vi "niRFUtil MASMT Util Constrained Linear Fit (SGL).vi"(0 "Y":sgl[](array[numeric]), 1 "method":i32(ring) items=["Least Square", "Least Absolute Residual", "Bisquare"], 5 "X":sgl[](array[numeric]), 7 "Weight":sgl[](array[numeric]), 9 "tolerance":sgl=0.0001, 11 "error in (no error)":errorcluster, 12 "parameter bounds":T1={"slope min"=-inf, "slope max"=inf, "intercept min"=-inf, "intercept max"=inf}) -> (4 "Best Linear Fit":sgl[](array[numeric]), 6 "slope":sgl, 8 "intercept":sgl, 10 "residue":sgl, 15 "error out":errorcluster)   [LabVIEW 2015, in "niRFUtil.lvlib"]
uses:
  niRFUtil.lvlib
  <vilib>/Analysis/NI_AALPro.lvlib
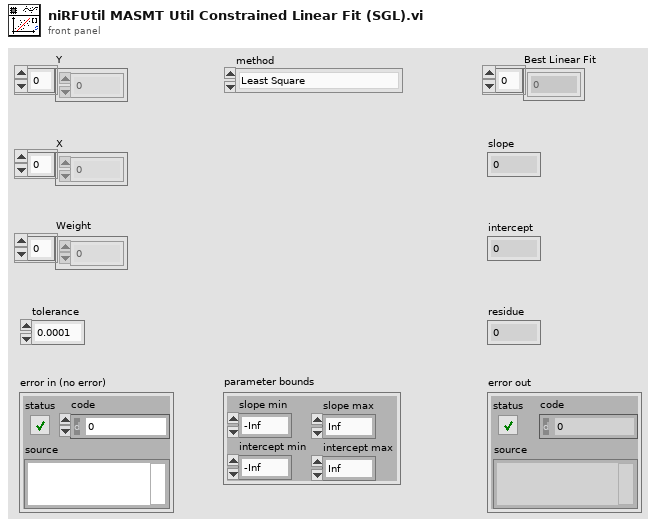
[diagram p1: front panel]
types:
  T1 = cluster{"slope min":sgl, "slope max":sgl, "intercept min":sgl, "intercept max":sgl}
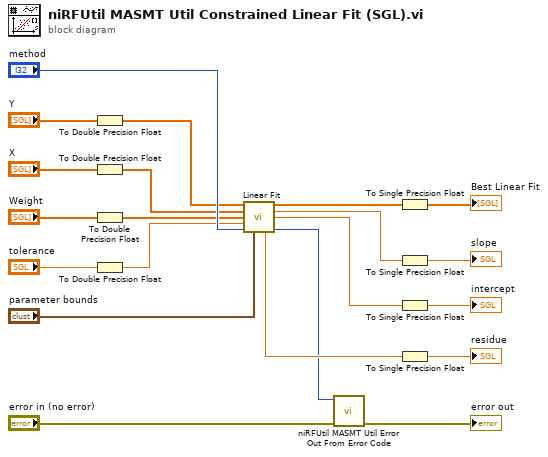
[diagram p0: block diagram]
diagram:
  n1 = To Double Precision Float(number="Y") -> (double precision float=w8:dbl[])
  n2 = To Double Precision Float(number="X") -> (double precision float=w7:dbl[])
  n3 = To Double Precision Float(number="Weight") -> (double precision float=w6:dbl[])
  n4 = To Double Precision Float(number="tolerance") -> (double precision float=w5:dbl)
  n5 = call <vilib>:"Linear Fit.vi"("Y"=w8, "X"=w7, "Weight"=w6, "tolerance"=w5, "method"="method", "parameter bounds"="parameter bounds") -> ("Best Linear Fit"=w20:dbl[], "slope"=w19:dbl, "intercept"=w18:dbl, "residue"=w17:dbl, "error"=w10:i32)  [unwired: 5 in]
  n6 = call "niRFUtil MASMT Util Error Out From Error Code.vi"("error in (no error)"="error in (no error)", "error code"=w10) -> ("error out"=→"error out":errorcluster)  [unwired: 9 in]
  n7 = To Single Precision Float(number=w20) -> (single precision float=→"Best Linear Fit":sgl[])
  n8 = To Single Precision Float(number=w19) -> (single precision float=→"slope":sgl)
  n9 = To Single Precision Float(number=w18) -> (single precision float=→"intercept":sgl)
  n10 = To Single Precision Float(number=w17) -> (single precision float=→"residue":sgl)
